vi "SwervePowerMath.vi"(6 "Turning?":bool, 8 "Turn_y":dbl, 9 "Turn_x":dbl, 10 "Lateral_y":dbl, 11 "Lateral_x":dbl) -> (0 "RRDrive":dbl, 1 "RLDrive":dbl, 2 "FRDrive":dbl, 3 "FLDrive":dbl)   [LabVIEW 2018]
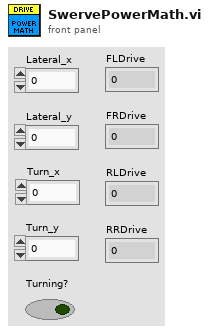
[diagram p1: front panel]
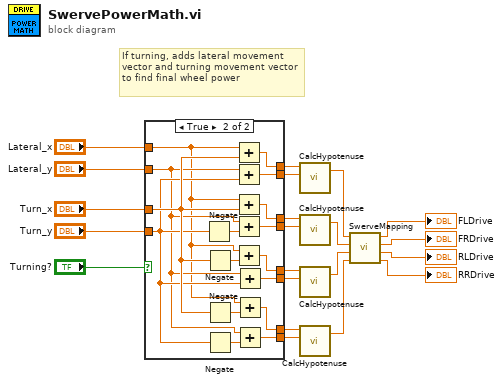
[diagram p0: block diagram]
diagram:
  # "If turning, adds lateral movement vector and turning movement vector to find final wheel power"
  n1 = case shown="True" "Turning?" {
    tunnel: [w23 w39] -> w21
    tunnel: [w22 w38] -> w20
    tunnel: [w23 w37] -> w19
    tunnel: [w22 w36] -> w18
    tunnel: [w23 w35] -> w17
    tunnel: [w22 w34] -> w16
    tunnel: [w23 w33] -> w15
    tunnel: [w22 w32] -> w14
    tunnel: "Turn_x" -> [_ w31]
    tunnel: "Turn_y" -> [_ w30]
    tunnel: "Lateral_y" -> [w23 w29]
    tunnel: "Lateral_x" -> [w22 w28]
    frame False {
    }
    frame True {
      n2 = Negate(x=w30) -> (-x=w27:dbl)
      n3 = Negate(x=w31) -> (-x=w26:dbl)
      n4 = Negate(x=w31) -> (-x=w24:dbl)
      n5 = Negate(x=w30) -> (-x=w25:dbl)
      n6 = Add(x=w28, y=w31) -> (x+y=w32:dbl)
      n7 = Add(x=w29, y=w30) -> (x+y=w33:dbl)
      n8 = Add(x=w28, y=w31) -> (x+y=w34:dbl)
      n9 = Add(x=w29, y=w27) -> (x+y=w35:dbl)
      n10 = Add(x=w28, y=w26) -> (x+y=w36:dbl)
      n11 = Add(x=w29, y=w30) -> (x+y=w37:dbl)
      n12 = Add(x=w28, y=w24) -> (x+y=w38:dbl)
      n13 = Add(x=w29, y=w25) -> (x+y=w39:dbl)
    }
  }
  n14 = call "CalcHypotenuse.vi"("b"=w15, "a"=w14) -> ("hypotenuse"=w9:dbl)  [unwired: 3 in]
  n15 = call "CalcHypotenuse.vi"("b"=w17, "a"=w16) -> ("hypotenuse"=w8:dbl)  [unwired: 3 in]
  n16 = call "CalcHypotenuse.vi"("b"=w19, "a"=w18) -> ("hypotenuse"=w7:dbl)  [unwired: 3 in]
  n17 = call "CalcHypotenuse.vi"("b"=w21, "a"=w20) -> ("hypotenuse"=w6:dbl)  [unwired: 3 in]
  n18 = call "SwerveMapping.vi"("RearRightDriveIn"=w6, "RearLeftDriveIn"=w7, "FrontRightDriveIn"=w8, "FrontLeftDriveIn"=w9) -> ("RearRightDriveOut"=→"RRDrive":dbl, "RearLeftDriveOut"=→"RLDrive":dbl, "FrontRightDriveOut"=→"FRDrive":dbl, "FrontLeftDriveOut"=→"FLDrive":dbl)  [unwired: 4 in]
